vi "Untitled 4.vi"() -> ()   [LabVIEW 2016]
uses:
  <vilib>/Instr/_visa.llb/VISA Configure Serial Port (Instr).vi
panel:
  out "read buffer":string
  in  "error in (no error)":errorcluster
  in  "VISA resource name":refnum<visa-resource-name>="COM4"
  in  "baud rate":u32=1500000
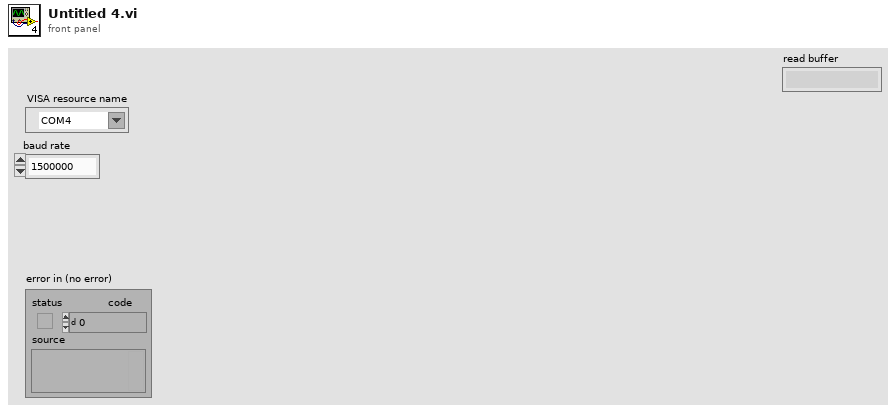
[diagram p1: front panel]
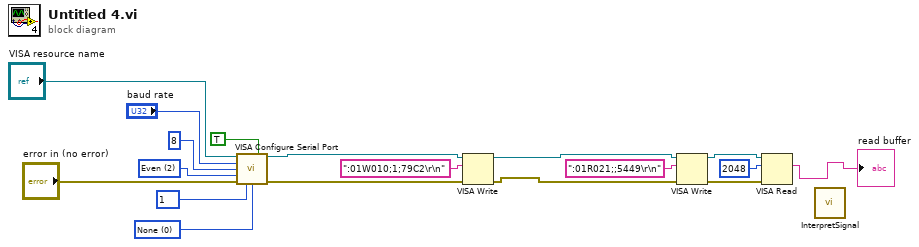
[diagram p0: block diagram]
diagram:
  w18 = u16 0 items=["None"=0, "XON/XOFF"=1, "RTS/CTS"=2, "DTR/DSR"=4] ("flow control")
  w17 = u16 10 items=["1"=10, "1.5"=15, "2.0"=20] ("stop bits")
  w16 = u16 2 items=["None", "Odd", "Even", "Mark", "Space"] ("parity")
  n1 = call-poly "VISA Configure Serial Port"("VISA resource name"="VISA resource name", "Enable Termination\nChar (T)"=TRUE, "baud rate (9600)"="baud rate", "data bits (8)"=u16 8 ("data bits"), "parity (0:none)"=w16, "error in (no error)"="error in (no error)", "stop bits (10: 1 bit)"=w17, "flow control (0:none)"=w18) -> ("VISA resource name out"=w5:refnum<visa-resource-name>, "error out"=w4:errorcluster)  [unwired: 6 in]
  n2 = VISA Write(VISA resource name=w5, write buffer=":01W010;1;79C2\r\n", error in (no error)=w4) -> (VISA resource name out=w3:refnum<visa-resource-name>, error out=w2:errorcluster)  [unwired: 1 out]
  n3 = VISA Write(VISA resource name=w3, write buffer=":01R021;;5449\r\n" ("Command"), error in (no error)=w2) -> (VISA resource name out=w9:refnum<visa-resource-name>, error out=w7:errorcluster)  [unwired: 1 out]
  n4 = VISA Read(VISA resource name=w9, byte count=u32 2048, error in (no error)=w7) -> (read buffer=→"read buffer":string)  [unwired: 3 out]
  n5 = call "InterpretSignal.vi"() -> ()  [unwired: 1 in, 1 out]
